vi "Multi-Graph Init.vi"(3 "Container State":T3, 4 "Previous State":variant, 5 "Previous Version":T2) -> (2 "Current State":T1)   [LabVIEW 2009, in "Multi-Graph.xctl"]
doc: "Demonstration of an XControl.\n\nAAL 9/09"
uses:
  Multi-Graph.xctl
  Multi-Graph State.ctl
  <vilib>/_xctls/Container State.ctl
  <vilib>/_xctls/Version.ctl
  <vilib>/_xctls/XControlSupport.lvlib
panel:
  in  "Default Indicator State":T1
  in  "Default Control State":T1
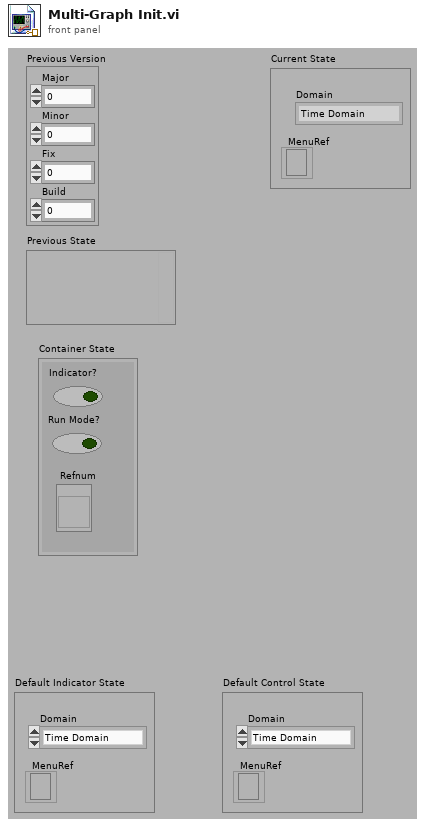
[diagram p1: front panel]
types:
  T1 = typedef "Multi-Graph.xctl/Multi-Graph State.ctl" = cluster{"Domain":enum16{"Time Domain", "Frequency Domain"}, "MenuRef":refnum<k9>}
  T2 = typedef "XControlSupport.lvlib/Version.ctl" = cluster{"Major":u16, "Minor":u16, "Fix":u16, "Build":u16}
  T3 = typedef "XControlSupport.lvlib/Container State.ctl" = cluster{"Indicator?":bool, "Run Mode?":bool, " Refnum":refnum<vi>}
  T4 = cluster{"Major":u16, "Minor":u16, "Fix":u16, "Build":u16}
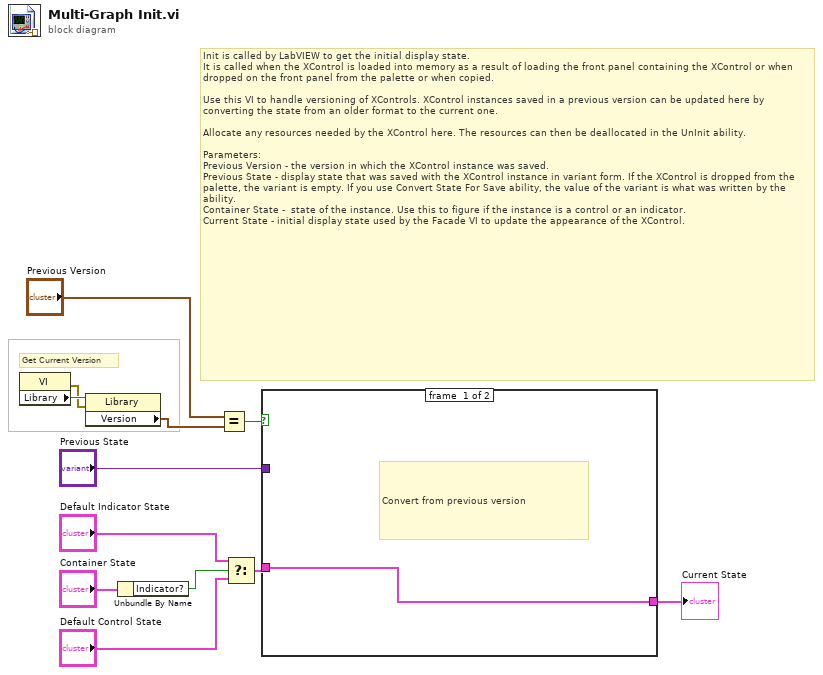
[diagram p0: block diagram]
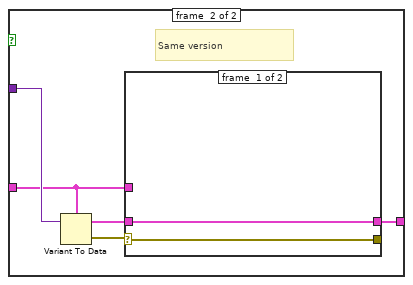
[diagram p2: hidden frame]
diagram:
  # "Get Current Version"
  # "Init is called by LabVIEW to get the initial display state.\nIt is called when the XControl is loaded into memory as a result of loading the front panel containing the XControl or when dropped on the front panel from the palette or when copied.\n\nUse this VI to handle versioning of XControls. XControl instances saved in a previous version can be updated here by converting the state from an older format to the current one.\n\nAllocate any resources needed by the XControl here. The resources can then be deallocated in the UnInit ability.\n\nParameters:\nPrevious Version - the version in which the XControl instance was saved.\nPrevious State - display state that was saved with the XControl instance in variant form. If the XControl is dropped from the palette, the variant is empty. If you use Convert State For Save ability, the value of the variant is what was written by the ability. \nContainer State -  state of the instance. Use this to figure if the instance is a control or an indicator.\nCurrent State - initial display state used by the Facade VI to update the appearance of the XControl."
  n1 = property class="VI"() -> (error out=w2:errorcluster, "Library"=w3:refnum<vi>)  [unwired: 2 in, 1 out]
  n2 = property class="Library"(reference=w3, error in=w2) -> ("Version"=w1:T4)  [unwired: 2 out]
  n3 = Unbundle By Name("Container State") -> ("Indicator?"=w5:bool)
  n4 = Equal?(x="Previous Version", y=w1) -> (x = y?=w11:bool)
  n5 = Select(t="Default Indicator State", s=w5, f="Default Control State") -> (s? t:f=w4:T1)
  n6 = case shown="True" w11 {
    tunnel: "Previous State" -> [_ w18]
    tunnel: [w13 w14] -> w9
    tunnel: w4 -> [w13 w15]
    frame #0 {
      # "Convert from previous version"
    }
    frame #1 {
      # "Same version"
      n7 = Variant To Data(Variant=w18, type=w15) -> (error out=w17:errorcluster, data=w16:T1)  [unwired: 1 in]
      n8 = case shown="Error" w17 {
        selector: w17 -> [w20 w21]
        tunnel: w16 -> [w19 _]
        tunnel: [w19 w22] -> w14
        tunnel: w15 -> [_ w22]
        tunnel: [w20 w21] -> _
        frame #0 {
        }
        frame #1 {
          # "Error converting previously \nsaved state. Use default instead."
        }
      }
    }
  }
  "Current State" <- w9
